vi "Set Icon Body Text.vi"() -> ()   [LabVIEW 2012]
uses:
  <vilib>/LabVIEW Icon API/lv_icon/Controls/Font.ctl
  <vilib>/LabVIEW Icon API/lv_icon/Classes/Icon/Icon.lvclass
  <vilib>/LabVIEW Icon API/lv_icon/Classes/Icon Framework/Icon Framework.lvclass
  <vilib>/LabVIEW Icon API/LabVIEW Icon API.lvlib
panel:
  out "Array":string[](array[string])
  in  "Body Text Spec.Size":u8
  in  "Body Text Spec.Font":T1
  in  "Class Path":path
  in  "Host":bool=TRUE
  in  "Project Path":path
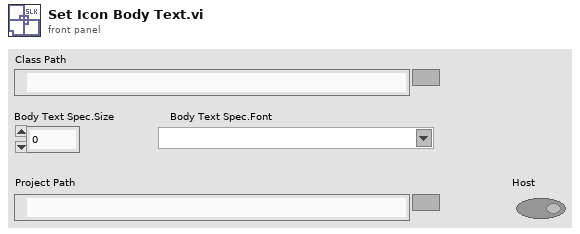
[diagram p1: front panel]
types:
  T1 = typedef "Font.ctl" = string
  T2 = typedef "BodyText.ctl" = cluster{"Line 1 text":string, "Line 2 text":string, "Line 3 text":string, "Line 4 text":string, "Line 1 color":u32, "Line 2 color":u32, "Line 3 color":u32, "Line 4 color":u32, "Body Text Spec":cluster{"Font":T1, "Alignment":T3, "Size":u8}, "Center text vertically":bool, "Capitalize Text":bool}
  T3 = typedef "Alignment.ctl" = u16
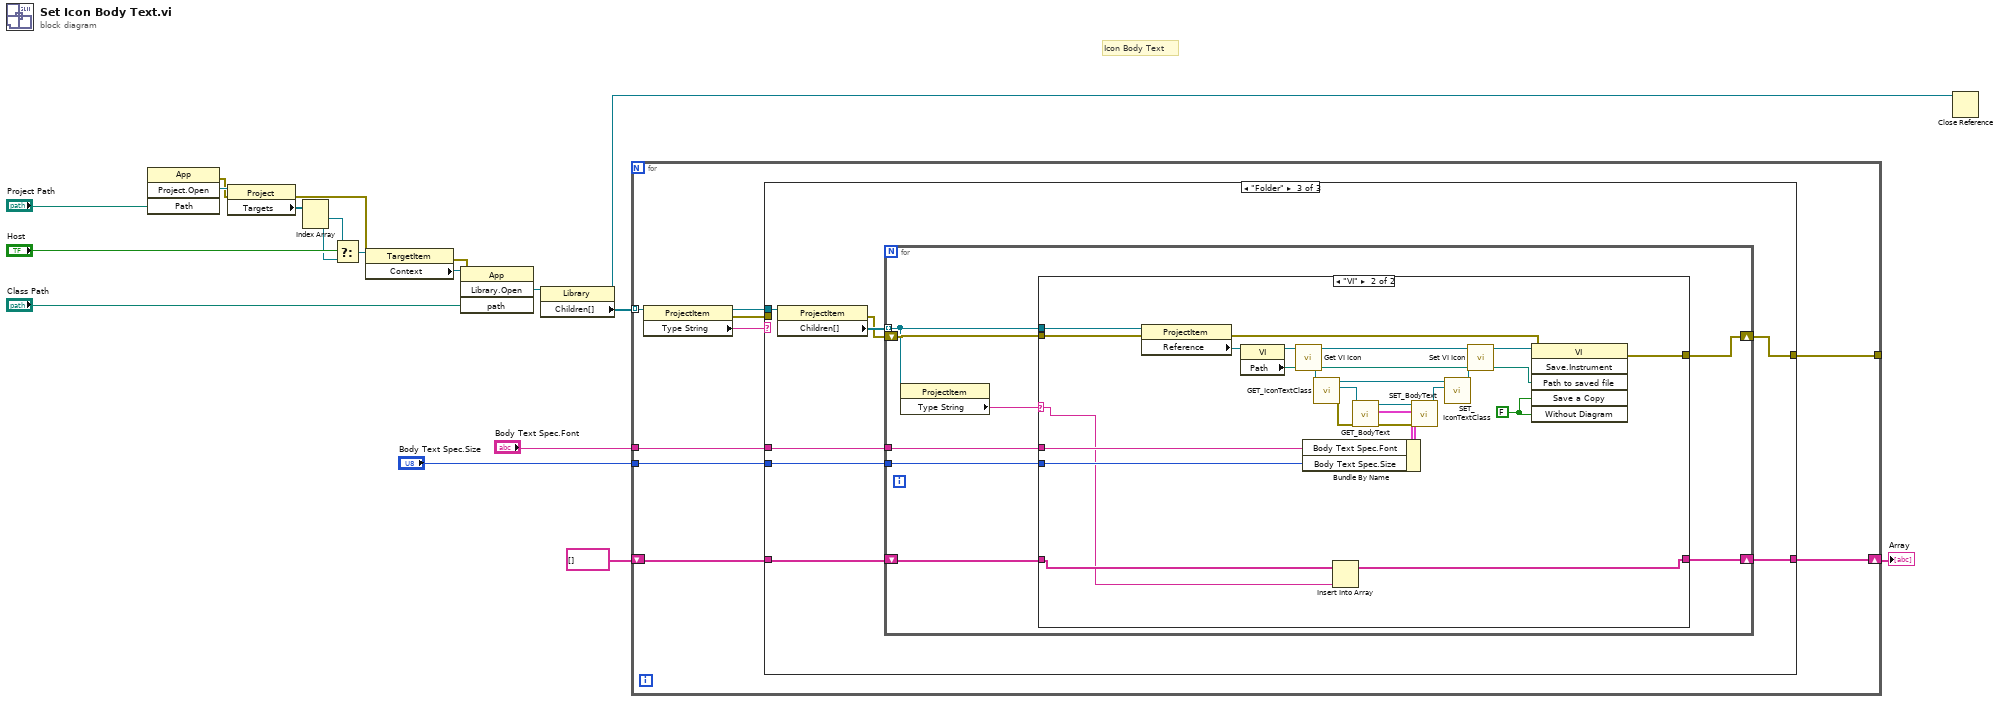
[diagram p0: block diagram]
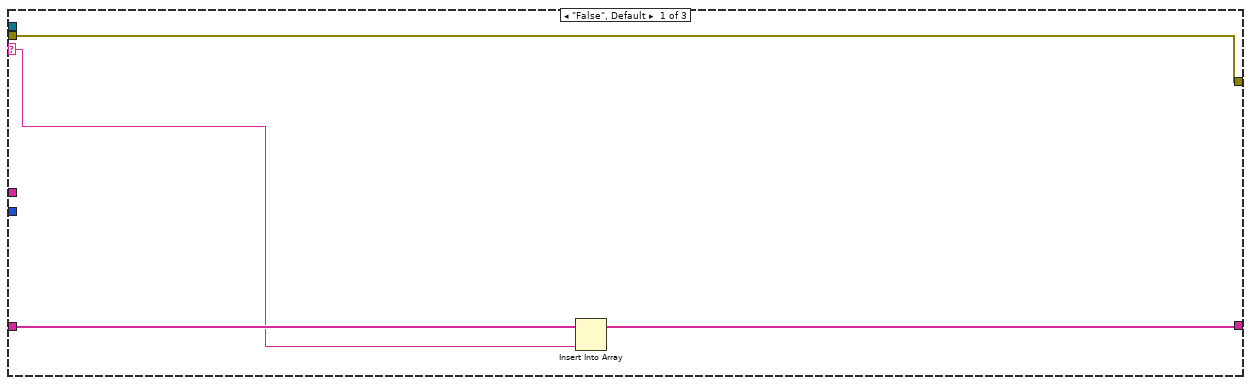
[diagram p2: hidden frame]
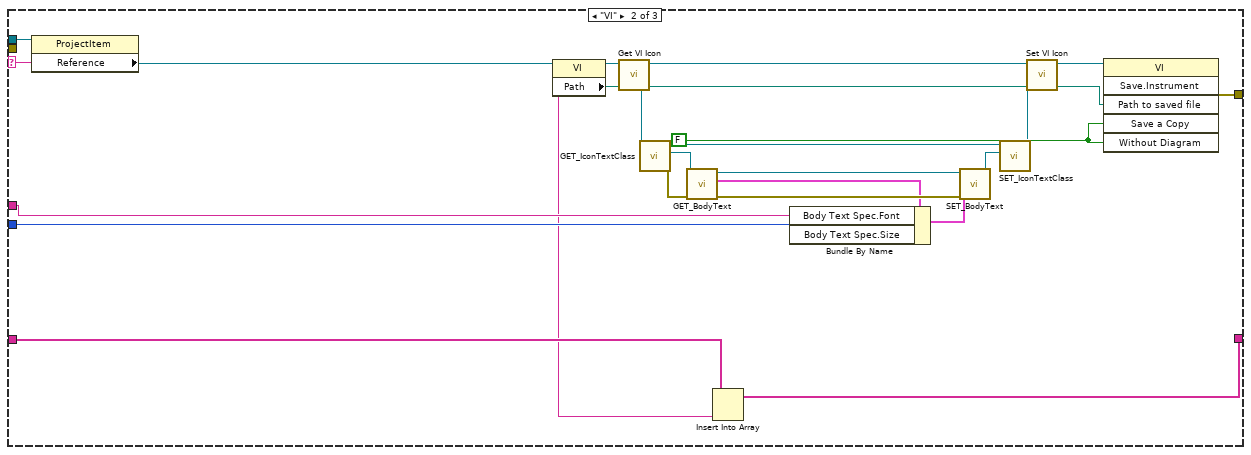
[diagram p3: hidden frame]
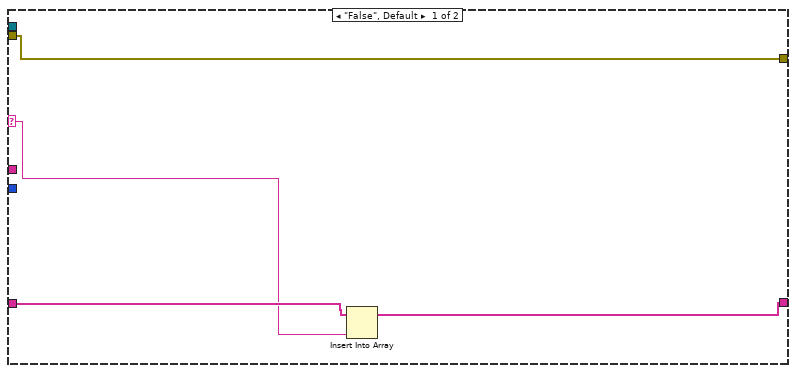
[diagram p4: hidden frame]
diagram:
  # "Icon Body Text"
  n1 = invoke class="App" method="Project.Open"("Path"="Project Path") -> (error out=w11:errorcluster, "Project:Open"=w18:refnum<vi>)  [unwired: 3 in, 2 out]
  n2 = property class="Project"(reference=w18, error in=w11) -> (error out=w10:errorcluster, "Targets"=w17:refnum<vi>[])  [unwired: 1 out]
  n3 = Index Array(array=w17) -> (element #1=w15:refnum<vi>, element #2=w14:refnum<vi>)  [unwired: 2 in]
  n4 = Select(t=w15, s="Host", f=w14) -> (s? t:f=w13:refnum<vi>)
  n5 = property class="TargetItem"(reference=w13, error in=w10) -> (error out=w9:errorcluster, "Context"=w5:refnum<vi>)  [unwired: 1 out]
  n6 = invoke class="App" method="Library.Open"(reference=w5, error in=w9, "path"="Class Path") -> ("Open Library"=w6:refnum<vi>)  [unwired: 1 in, 3 out]
  n7 = property class="Library"(reference=w6) -> (reference out=w7:refnum<vi>, "Children[]"=w8:refnum<vi>[])  [unwired: 1 in, 1 out]
  n8 = for {
    tunnel: w8 -> [w28] mode=indexing
    tunnel: [w25] -> _
    tunnel: "Body Text Spec.Font" -> [w23]
    tunnel: "Body Text Spec.Size" -> [w22]
    shift-right: [w21] -> w1
    shift-left: string[] [] -> [w20]
    n9 = property class="ProjectItem"(reference=w28) -> (reference out=w27:refnum<vi>, error out=w24:errorcluster, "Type String"=w26:string)  [unwired: 1 in]
    n10 = case shown="\"Folder\"" w26 {
      selector: w26 -> [w29 w33 _]
      tunnel: w27 -> [_ w55 w63]
      tunnel: [w32 w40 w61] -> w25
      tunnel: w24 -> [w32 _ _]
      tunnel: w23 -> [_ w37 w59]
      tunnel: w22 -> [_ w36 w58]
      tunnel: [w30 w35 w57] -> w21
      tunnel: w20 -> [w31 w34 w56]
      frame "False", Default {
        n11 = Insert Into Array(array=w31, new element=w29) -> (w30:string[])  [unwired: 1 in]
      }
      frame "VI" {
        w54 = FALSE ("Save a Copy")
        n12 = property class="ProjectItem"(reference=w55) -> ("Reference"=w43:refnum<vi>)  [unwired: 1 in, 2 out]
        n13 = property class="VI"(reference=w43) -> (reference out=w41:refnum<vi>, "Path"=w42:path)  [unwired: 1 in, 1 out]
        n14 = call <vilib>:"Get VI Icon.vi"("VI Refnum in"=w41) -> ("Icon"=w53:refnum<class "Icon.lvclass">, "VI Refnum out"=w46:refnum<vi>)  [unwired: 8 in, 1 out]
        n15 = call-dynamic "GET_IconTextClass.vi"("Icon.lvclass in"=w53) -> ("error out"=w47:errorcluster, "Icon Framework.lvclass"=w52:refnum<class "Icon Framework.lvclass">, "Icon.lvclass out"=w50:refnum<class "Icon.lvclass">)  [unwired: 8 in]
        n16 = call-dynamic "GET_BodyText.vi"("error in (no error)"=w47, "Icon Framework.lvclass in"=w52) -> ("error out"=w48:errorcluster, "Body Text"=w39:T2, "Icon Framework.lvclass out"=w51:refnum<class "Icon Framework.lvclass">)  [unwired: 6 in, 1 out]
        n17 = Insert Into Array(array=w34, new element=w33) -> (w35:string[])  [unwired: 1 in]
        n18 = Bundle By Name(cluster=w39, "Body Text Spec.Font"=w37, "Body Text Spec.Size"=w36) -> (w38:T2)
        n19 = call-dynamic "SET_BodyText.vi"("error in (no error)"=w48, "Body Text"=w38, "Icon Framework.lvclass in"=w51) -> ("Icon Framework.lvclass out"=w49:refnum<class "Icon Framework.lvclass">)  [unwired: 7 in, 1 out]
        n20 = call-dynamic "SET_IconTextClass.vi"("Icon Framework.lvclass"=w49, "Icon.lvclass in"=w50) -> ("Icon.lvclass out"=w45:refnum<class "Icon.lvclass">)  [unwired: 8 in, 1 out]
        n21 = call <vilib>:"Set VI Icon.vi"("Icon"=w45, "VI Refnum in"=w46) -> ("VI Refnum out"=w44:refnum<vi>)  [unwired: 8 in, 1 out]
        n22 = invoke class="VI" method="Save.Instrument"(reference=w44, "Path to saved file"=w42, "Save a Copy"=w54, "Without Diagram"=w54) -> (error out=w40:errorcluster)  [unwired: 2 in, 5 out]
      }
      frame "Folder" {
        n23 = property class="ProjectItem"(reference=w63) -> (error out=w60:errorcluster, "Children[]"=w62:refnum<vi>[])  [unwired: 1 in, 1 out]
        n24 = for {
          tunnel: w62 -> [w67] mode=indexing
          shift-right: [w71] -> w61
          shift-left: w60 -> [w70]
          tunnel: w59 -> [w69]
          tunnel: w58 -> [w68]
          shift-right: [w65] -> w57
          shift-left: w56 -> [w64]
          n25 = property class="ProjectItem"(reference=w67) -> ("Type String"=w66:string)  [unwired: 1 in, 2 out]
          n26 = case shown="\"VI\"" w66 {
            selector: w66 -> [w72 w76]
            tunnel: w67 -> [_ w86]
            tunnel: [w75 w85] -> w71
            tunnel: w70 -> [w75 w84]
            tunnel: w69 -> [_ w80]
            tunnel: w68 -> [_ w79]
            tunnel: [w73 w77] -> w65
            tunnel: w64 -> [w74 w78]
            frame "False", Default {
              n27 = Insert Into Array(array=w74, new element=w72) -> (w73:string[])  [unwired: 1 in]
            }
            frame "VI" {
              w100 = FALSE ("Save a Copy")
              n28 = property class="ProjectItem"(reference=w86, error in=w84) -> (error out=w83:errorcluster, "Reference"=w89:refnum<vi>)  [unwired: 1 out]
              n29 = property class="VI"(reference=w89) -> (reference out=w87:refnum<vi>, "Path"=w88:path)  [unwired: 1 in, 1 out]
              n30 = call <vilib>:"Get VI Icon.vi"("VI Refnum in"=w87) -> ("Icon"=w99:refnum<class "Icon.lvclass">, "VI Refnum out"=w92:refnum<vi>)  [unwired: 8 in, 1 out]
              n31 = call-dynamic "GET_IconTextClass.vi"("Icon.lvclass in"=w99) -> ("error out"=w93:errorcluster, "Icon Framework.lvclass"=w98:refnum<class "Icon Framework.lvclass">, "Icon.lvclass out"=w96:refnum<class "Icon.lvclass">)  [unwired: 8 in]
              n32 = Insert Into Array(array=w78, new element=w76) -> (w77:string[])  [unwired: 1 in]
              n33 = call-dynamic "GET_BodyText.vi"("error in (no error)"=w93, "Icon Framework.lvclass in"=w98) -> ("error out"=w94:errorcluster, "Body Text"=w82:T2, "Icon Framework.lvclass out"=w97:refnum<class "Icon Framework.lvclass">)  [unwired: 6 in, 1 out]
              n34 = Bundle By Name(cluster=w82, "Body Text Spec.Font"=w80, "Body Text Spec.Size"=w79) -> (w81:T2)
              n35 = call-dynamic "SET_BodyText.vi"("error in (no error)"=w94, "Body Text"=w81, "Icon Framework.lvclass in"=w97) -> ("Icon Framework.lvclass out"=w95:refnum<class "Icon Framework.lvclass">)  [unwired: 7 in, 1 out]
              n36 = call-dynamic "SET_IconTextClass.vi"("Icon Framework.lvclass"=w95, "Icon.lvclass in"=w96) -> ("Icon.lvclass out"=w91:refnum<class "Icon.lvclass">)  [unwired: 8 in, 1 out]
              n37 = call <vilib>:"Set VI Icon.vi"("Icon"=w91, "VI Refnum in"=w92) -> ("VI Refnum out"=w90:refnum<vi>)  [unwired: 8 in, 1 out]
              n38 = invoke class="VI" method="Save.Instrument"(reference=w90, error in=w83, "Path to saved file"=w88, "Save a Copy"=w100, "Without Diagram"=w100) -> (error out=w85:errorcluster)  [unwired: 1 in, 5 out]
            }
          }
        }
      }
    }
  }
  "Array" <- w1
  n39 = Close Reference(reference=w7) -> ()  [unwired: 1 in, 1 out]
